vi "CheckSingleBitConnections.vi"(3 "error in (no error)":errorcluster, 4 "Connection ID CC":refnum<k5>, 5 "Chopper Serial Number":string="26", 6 "Connection ID TB":refnum<k5>) -> (0 "error out":errorcluster, 1 "PASS / FAIL":bool, 2 "RESULT":string)   [LabVIEW 2013]
panel:
  out "PROGRESS":i32(slide) scale=0.0..11.0
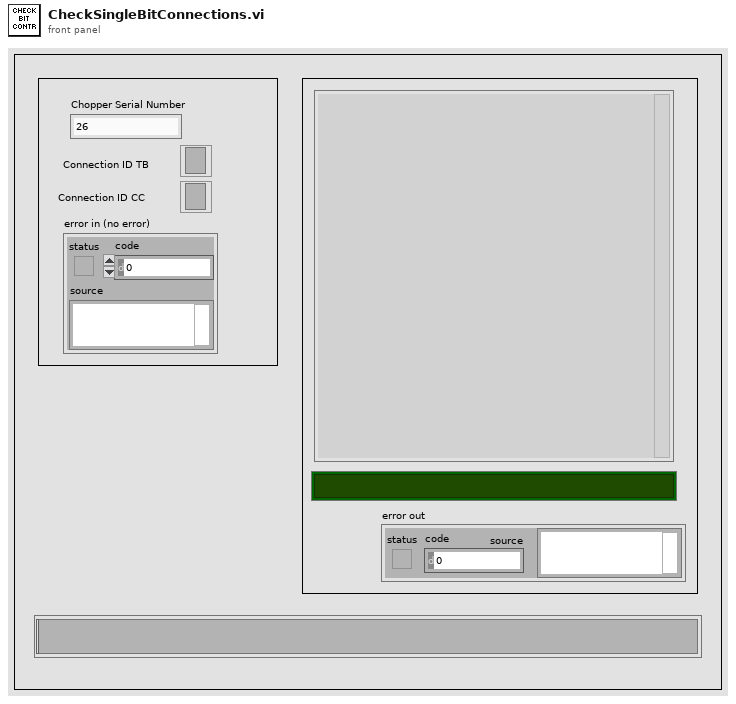
[diagram p1: front panel]
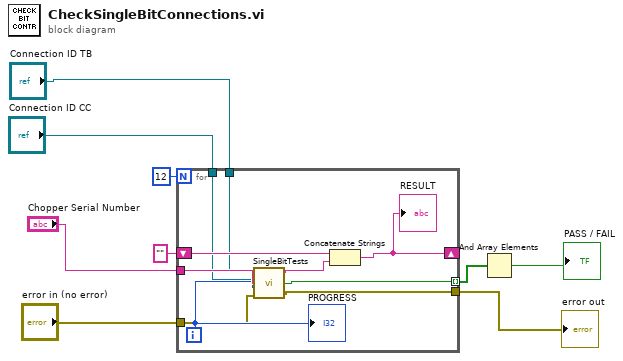
[diagram p0: block diagram]
diagram:
  n1 = for {
    N: 12 -> [_]
    shift-right: [w18] -> _
    shift-left: "" ("String") -> [w19]
    tunnel: "Chopper Serial Number" -> [w16]
    tunnel: "error in (no error)" -> [w14]
    tunnel: [w13] -> w7
    tunnel: [w12] -> w4 mode=indexing
    tunnel: "Connection ID CC" -> [w11]
    tunnel: "Connection ID TB" -> [w10]
    i -> [w15]
    n2 = call "SingleBitTests.vi"("Connection ID TB"=w10, "connection ID CC"=w11, "Ring"=w15, "error in (no error)"=w14, "Chopper Serial Number"=w16) -> ("String"=w17:string, "PASS"=w12:bool, "error out"=w13:errorcluster)
    n3 = Concatenate Strings(w19, w17) -> (w18:string)
    "RESULT" <- w18
    "PROGRESS" <- w15
  }
  "error out" <- w7
  n4 = And Array Elements(Boolean array=w4) -> (logical AND=→"PASS / FAIL":bool)
